vi "Activity log GUI.vi"(8 "error in (no error)":errorcluster, 10 "Use DITs? (T)":bool=TRUE, 11 "Activity Log Filepath In":path=path "C:/Project - VSS/Wellplate Inspection System/activity log.txt") -> (0 "error out":errorcluster, 3 "Activity Log Filepath Out":path=path "C:/Documents and Settings/default/Desktop/New Folder/passwords.log")   [LabVIEW 2009]
doc: "Reads the activity log at\"Activity log fiepath in\". Displays activities in a multicolumn listbox with a timestamp and activity description field."
uses:
  GUI/GUI.lvlib
panel:
  in  "Return":bool
  in  "DIT Key Info":T1
  out "Activity Log":i32[](listbox)
  out "Activity Log Path":path
  out "File Is Valid":bool
  out "DIT Text Found":bool
  # "checked = valid activity\nunchecked = not validated"
  # "Reverse order -most recent activities 1st in list"
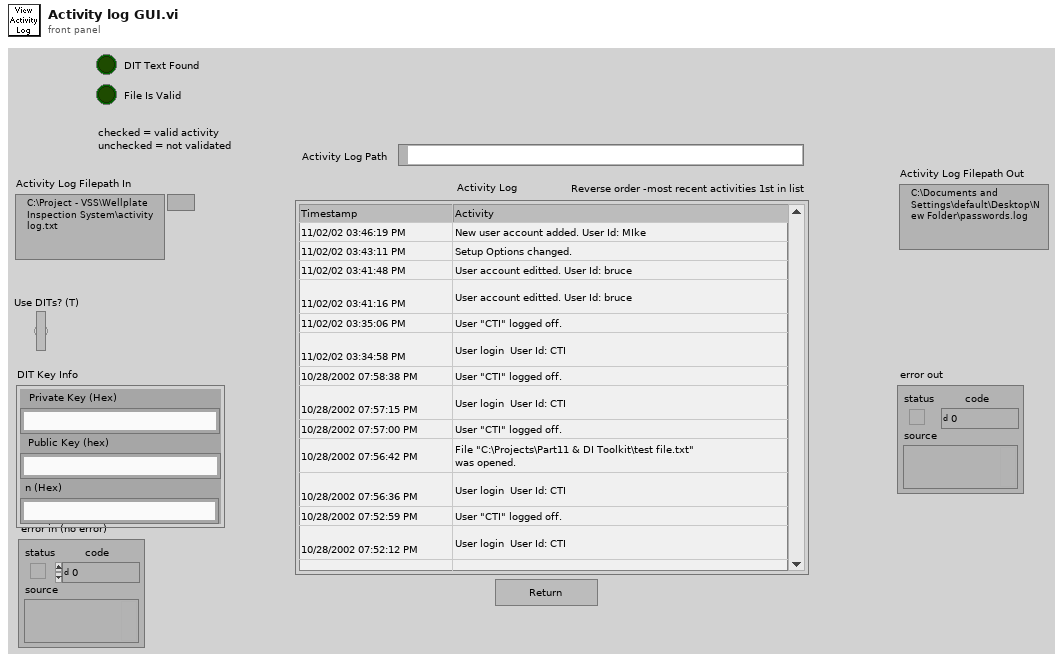
[diagram p1: front panel]
types:
  T1 = cluster{"Private Key (Hex)":string, "Public Key (hex)":string, "n (Hex)":string}
  T2 = cluster{"Date String":string, "Activity Log String":string}[]
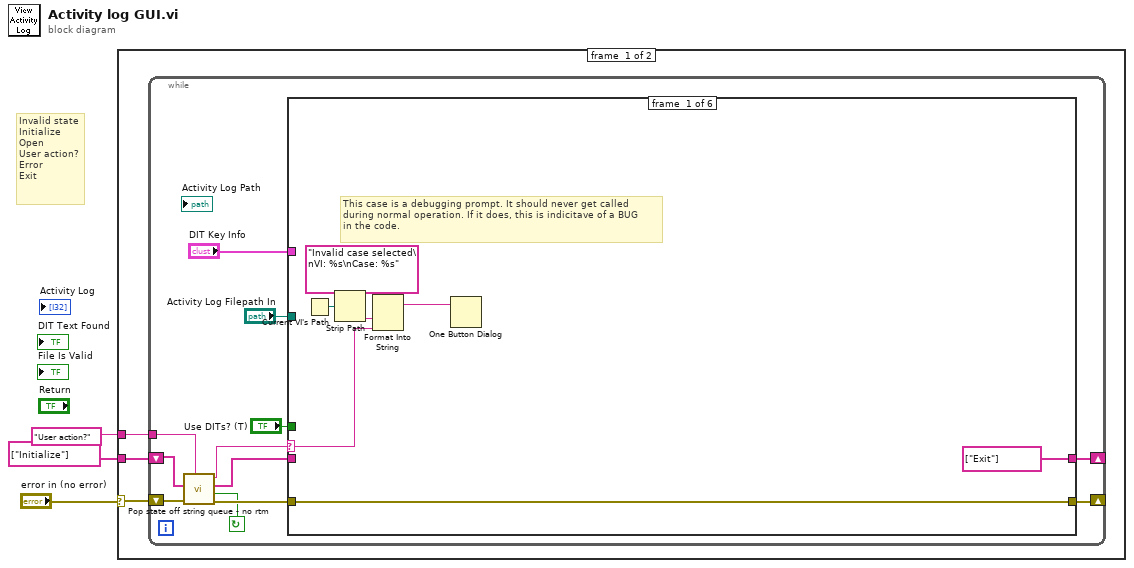
[diagram p0: block diagram]
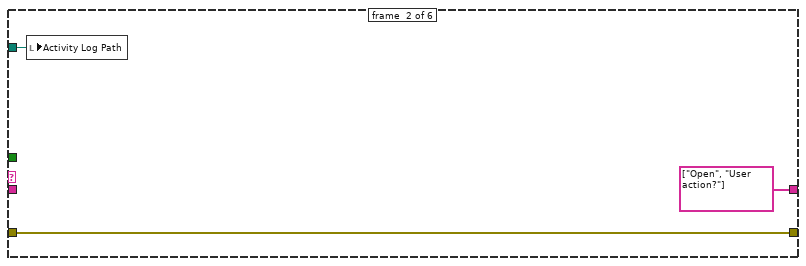
[diagram p2: hidden frame]
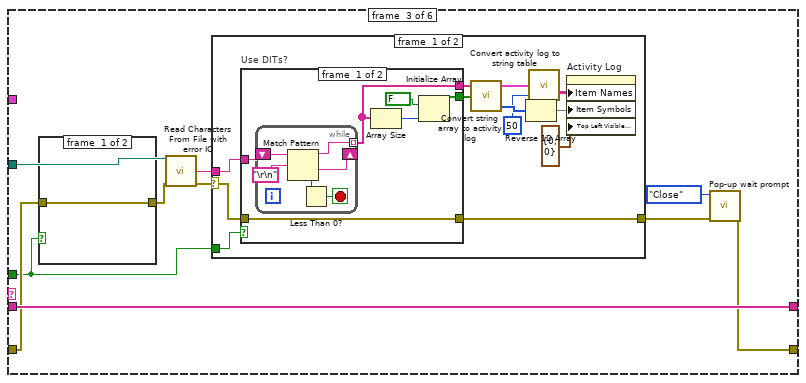
[diagram p3: hidden frame]
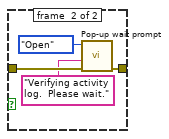
[diagram p4: hidden frame]
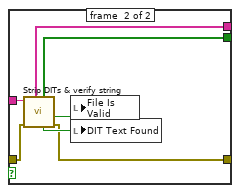
[diagram p5: hidden frame]
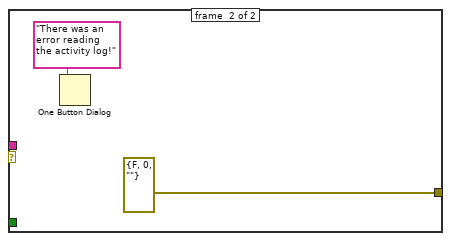
[diagram p6: hidden frame]
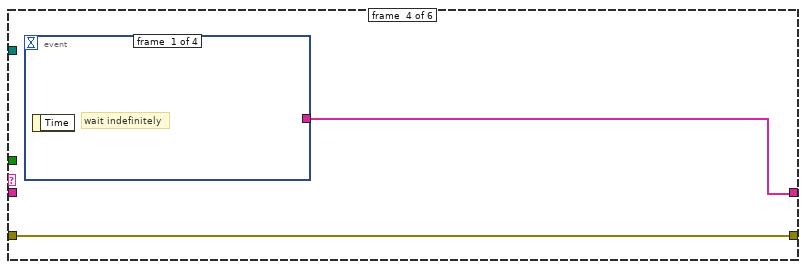
[diagram p7: hidden frame]
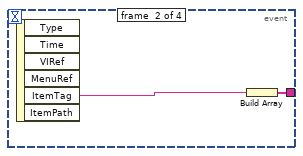
[diagram p8: hidden frame]
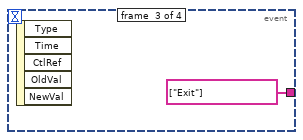
[diagram p9: hidden frame]
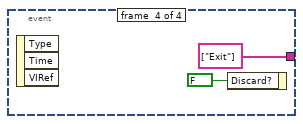
[diagram p10: hidden frame]
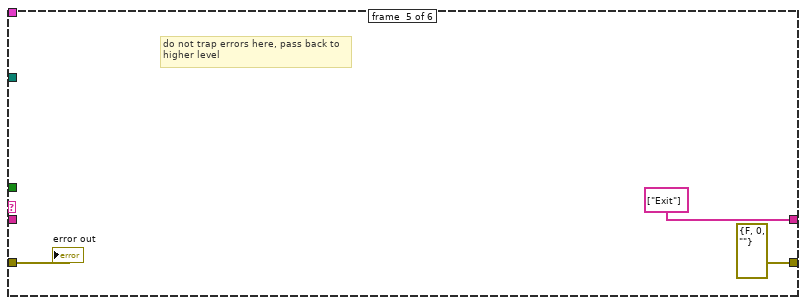
[diagram p11: hidden frame]
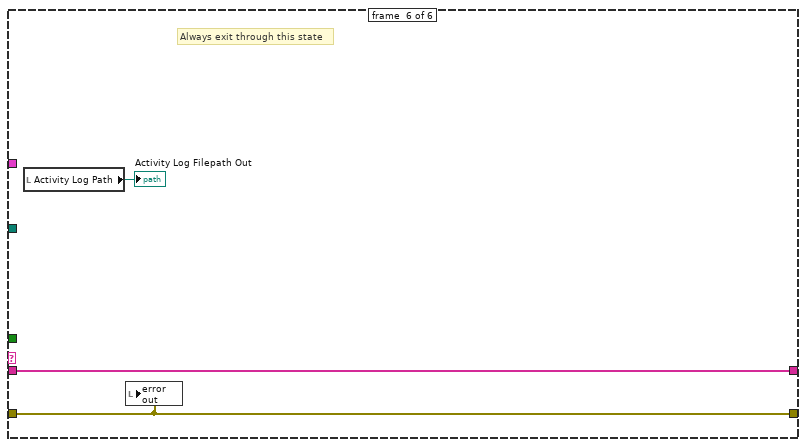
[diagram p12: hidden frame]
diagram:
  # "Invalid state\nInitialize\nOpen\nUser action?\nError\nExit"
  n1 = case shown="No Error" "error in (no error)" {
    selector: "error in (no error)" -> [w6 _]
    tunnel: string[] ["Initialize"] ("State que out") -> [w5 _]
    tunnel: "User action?" ("Default state") -> [w4 _]
    frame #0 {
      n2 = while {
        tunnel: w4 -> [w10]
        shift-left: w5 -> [w14]
        shift-right: [w12] -> _
        shift-left: w6 -> [w18]
        shift-right: [w16] -> _
        stop <- w11 continue-if-true
        n3 = call "Pop state off string queue - no rtm.vi"("Default state"=w10, "error in (no error)"=w18, "State que in"=w14) -> ("error out"=w17:errorcluster, "Not Exit?"=w11:bool, "State que out"=w13:string[], "State case"=w15:string)  [unwired: 5 out]
        n4 = case shown="\"Open\"" w15 {
          selector: w15 -> [w20 _ _ _ _ _]
          tunnel: [w25 w26 w31 w78 errorcluster {"status"=FALSE, "code"=0, "source"=""} ("error out") w88] -> w16
          tunnel: w17 -> [w25 w26 w33 w78 w84 w88]
          tunnel: [string[] ["Exit"] ("State que out") string[] ["Open", "User action?"] ("State que out") w38 w77 string[] ["Exit"] ("State que out") w89] -> w12
          tunnel: w13 -> [_ _ w38 _ _ w89]
          tunnel: "Activity Log Filepath In" -> [_ w28 w35 _ _ _]
          tunnel: "DIT Key Info" -> [_ _ _ _ _ _]
          tunnel: "Use DITs? (T)" -> [_ _ w29 _ _ _]
          frame #0 {
            # "This case is a debugging prompt. It should never get called\nduring normal operation. If it does, this is indicitave of a BUG\nin the code."
            n5 = Current VI's Path() -> (path=w22:path)
            n6 = Strip Path(path=w22) -> (name=w21:string)  [unwired: 1 out]
            n7 = Format Into String(format string="Invalid case selected\nVI: %s\nCase: %s" ("message"), w21, w20) -> (resulting string=w23:string)  [unwired: 2 in, 1 out]
            n8 = One Button Dialog(message=w23) -> ()  [unwired: 2 out]
          }
          frame #1 {
            n9 = local write "Activity Log Path"(w28) -> ()
          }
          frame #2 {
            n10 = case shown="True" w29 {
              tunnel: [w39 w43] -> w34
              tunnel: w33 -> [w39 w42]
              frame #0 {
              }
              frame #1 {
                n11 = call "Pop-up wait prompt.vi"("error in (no error)"=w42, "Prompt Text"="Verifying activity log.  Please wait.", "Control"=enum16{"Open", "Close", "Status", "No Change"}."Open") -> ("error out"=w43:errorcluster)  [unwired: 8 out]
              }
            }
            n12 = call "Read Characters From File with error IO.vi"("file path (dialog if empty)"=w35, "error in (no error)"=w34) -> ("character string"=w37:string, "error out"=w36:errorcluster)  [unwired: 3 in, 9 out]
            n13 = case shown="No Error" w36 {
              selector: w36 -> [w53 _]
              tunnel: [w55 errorcluster {"status"=FALSE, "code"=0, "source"=""} ("error out")] -> w32
              tunnel: w37 -> [w54 _]
              tunnel: w29 -> [w44 _]
              frame #0 {
                n14 = case "Use DITs?" shown="False" w44 {
                  tunnel: [w61 w72] -> w55
                  tunnel: w54 -> [w60 w71]
                  tunnel: w53 -> [w61 w70]
                  tunnel: [w59 w69] -> w51
                  tunnel: [w56 w68] -> w50
                  frame #0 {
                    n15 = while {
                      shift-right: [w65] -> _
                      shift-left: w60 -> [w67]
                      tunnel: [w66] -> w59 mode=indexing
                      stop <- w63 stop-if-true
                      n16 = Match Pattern(string=w67, regular expression="\r\n") -> (before substring=w66:string, after substring=w65:string, offset past match=w62:i32)  [unwired: 2 out]
                      n17 = Less Than 0?(x=w62) -> (x < 0?=w63:bool)
                    }
                    n18 = Array Size(array=w59) -> (size(s)=w58:i32)
                    n19 = Initialize Array(FALSE, w58) -> (w56:bool[])
                  }
                  frame #1 {
                    n20 = call "Strip DITs & verify string.vi"("error in (no error)"=w70, "Text & DIT(s)"=w71) -> ("error out"=w72:errorcluster, "DITs valid?"=w74:bool, "DIT(s) found?"=w73:bool, "Valid DITs array"=w68:bool[], "Text array"=w69:string[])  [unwired: 5 out]
                    n21 = local write "File Is Valid"(w74) -> ()
                    n22 = local write "DIT Text Found"(w73) -> ()
                  }
                }
                n23 = call "Convert string array to activity log.vi"("Valid DITs Array"=w50, "Activity Log String Array"=w51) -> ("Activity Log Valid? symbols array"=w49:i32[], "Activity Array"=w48:T2)  [unwired: 1 in, 1 out]
                n24 = Reverse 1D Array(array=w49) -> (reversed array=w45:i32[])
                n25 = call "Convert activity log to string table.vi"("Chars per line"=u8 50, "Activity Array"=w48) -> ("Table"=w52:string[][])  [unwired: 3 out]
                n26 = property on="Activity Log" class="MCListbox (strict)"("Item Names"=w52, "Item Symbols"=w45, "Top Left Visible Cell"=cluster{u32, u32} {0, 0}) -> ()  [unwired: 2 in, 2 out]
              }
              frame #1 {
                n27 = One Button Dialog(message="There was an error reading the activity log!") -> ()  [unwired: 2 out]
              }
            }
            n28 = call "Pop-up wait prompt.vi"("error in (no error)"=w32, "Control"=enum16{"Open", "Close", "Status", "No Change"}."Close") -> ("error out"=w31:errorcluster)  [unwired: 1 in, 8 out]
          }
          frame #3 {
            n29 = event shown="[2] \"Return\": Value Change" {
              selector: _ -> [_ _ _ _]
              dyn-events: _ -> [_ _ _ _]
              timeout: _ -> [_ _ _ _]
              tunnel: [_ w79 string[] ["Exit"] ("State que out") string[] ["Exit"] ("State que out")] -> w77
              event #0 {
                # "wait indefinitely"
                n30 = event-data() -> ()  [unwired: 2 out]
              }
              event #1 {
                n31 = event-data() -> ("ItemTag"=w80:string)  [unwired: 6 out]
                n32 = Build Array(w80) -> (w79:string[])
              }
              event #2 {
                n33 = event-data() -> ()  [unwired: 6 out]
              }
              event #3 {
                n34 = event-data() -> ()  [unwired: 4 out]
                n35 = event-data("Discard?"=FALSE) -> ()  [unwired: 1 in, 1 out]
              }
            }
          }
          frame #4 {
            # "do not trap errors here, pass back to\nhigher level"
            "error out" <- w84
          }
          frame #5 {
            # "Always exit through this state"
            n36 = local read "Activity Log Path"() -> (→"Activity Log Filepath Out":path)
            n37 = local write "error out"(w88) -> ()
          }
        }
      }
    }
    frame #1 {
    }
  }
